vi "Creat Init Files.vi"(8 "error in (no error)":errorcluster, 11 "Setup File in":refnum<class "Setup File.lvclass">) -> (0 "error out":errorcluster, 3 "Setup File out":refnum<class "Setup File.lvclass">)   [LabVIEW 2018, in "Setup File.lvclass"]
doc: "Este VI cria uma pasta chamada Setup File que contém os seguintes arquivos de pré-configuração das câmeras: Bias, Comparação, Flat Field, Slow Acquisition, Normal Acquisition e Fast Acquisition."
uses:
  Setup File.lvclass
  Setup File.lvclass/Setup File.ctl
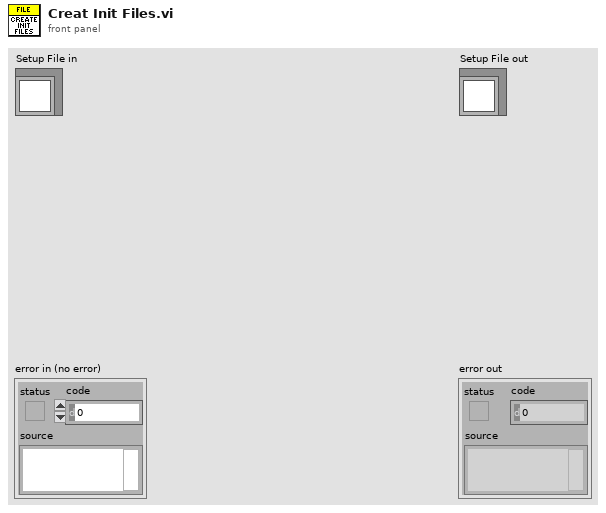
[diagram p1: front panel]
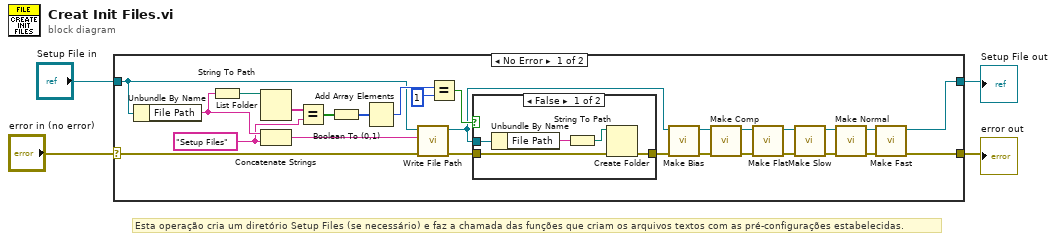
[diagram p0: block diagram]
diagram:
  # "Esta operação cria um diretório Setup Files (se necessário) e faz a chamada das funções que criam os arquivos textos com as pré-configurações estabelecidas."
  n1 = case shown="No Error" "error in (no error)" {
    selector: "error in (no error)" -> [w23 w39]
    tunnel: [w5 w39] -> w3
    tunnel: [w6 w38] -> w1
    tunnel: "Setup File in" -> [w24 w38]
    frame No Error {
      w19 = "Setup Files"
      n2 = Unbundle By Name(w24) -> ("File Path"=w20:string)
      n3 = String To Path(string=w20) -> (path=w31:path)
      n4 = List Folder(path=w31) -> (folder names=w30:string[])  [unwired: 3 in, 3 out]
      n5 = Concatenate Strings(w20, w19) -> (w21:string)
      n6 = Equal?(x=w30, y=w19) -> (x = y?=w26:bool[])
      n7 = Boolean To (0,1)(Boolean=w26) -> (0, 1=w27:i16[])
      n8 = Add Array Elements(numeric array=w27) -> (sum=w28:i16)
      n9 = call "Write File Path.vi"("error in (no error)"=w23, "File Path"=w21, "Setup File in"=w24) -> ("error out"=w22:errorcluster, "Setup File out"=w14:refnum<class "Setup File.lvclass">)  [unwired: 7 in]
      n10 = Equal?(x=w28, y=i16 1) -> (x = y?=w25:bool)
      n11 = case shown="False" w25 {
        tunnel: w14 -> [w34 _]
        tunnel: w22 -> [w36 w37]
        tunnel: [w32 w37] -> w13
        frame False {
          n12 = Unbundle By Name(w34) -> ("File Path"=w33:string)
          n13 = String To Path(string=w33) -> (path=w35:path)
          n14 = Create Folder(path (use dialog)=w35, error in=w36) -> (error out=w32:errorcluster)  [unwired: 1 in, 2 out]
        }
        frame True {
        }
      }
      n15 = call "Make Bias.vi"("error in (no error)"=w13, "Setup File in"=w14) -> ("error out"=w15:errorcluster, "Setup File out"=w18:refnum<class "Setup File.lvclass">)  [unwired: 8 in]
      n16 = call "Make Comp.vi"("error in (no error)"=w15, "Setup File in"=w18) -> ("error out"=w16:errorcluster, "Setup File out"=w17:refnum<class "Setup File.lvclass">)  [unwired: 8 in]
      n17 = call "Make Flat.vi"("error in (no error)"=w16, "Setup File in"=w17) -> ("error out"=w10:errorcluster, "Setup File out"=w9:refnum<class "Setup File.lvclass">)  [unwired: 8 in]
      n18 = call "Make Slow.vi"("error in (no error)"=w10, "Setup File in"=w9) -> ("error out"=w11:errorcluster, "Setup File out"=w12:refnum<class "Setup File.lvclass">)  [unwired: 8 in]
      n19 = call "Make Normal.vi"("error in (no error)"=w11, "Setup File in"=w12) -> ("error out"=w8:errorcluster, "Setup File out"=w7:refnum<class "Setup File.lvclass">)  [unwired: 8 in]
      n20 = call "Make Fast.vi"("error in (no error)"=w8, "Setup File in"=w7) -> ("error out"=w5:errorcluster, "Setup File out"=w6:refnum<class "Setup File.lvclass">)  [unwired: 8 in]
    }
    frame Error {
    }
  }
  "error out" <- w3
  "Setup File out" <- w1
